vi "Read Action.vi"(8 "error in (no error)":errorcluster, 11 "Debug Data in":refnum<class "Debug Data.lvclass">) -> (0 "error out":errorcluster, 2 "Action":string, 3 "Debug Data out":refnum<class "Debug Data.lvclass">)   [LabVIEW 2020, in "Debug Data.lvclass"]
uses:
  Debug Data.lvclass
  Debug Data.lvclass/Debug Data.ctl
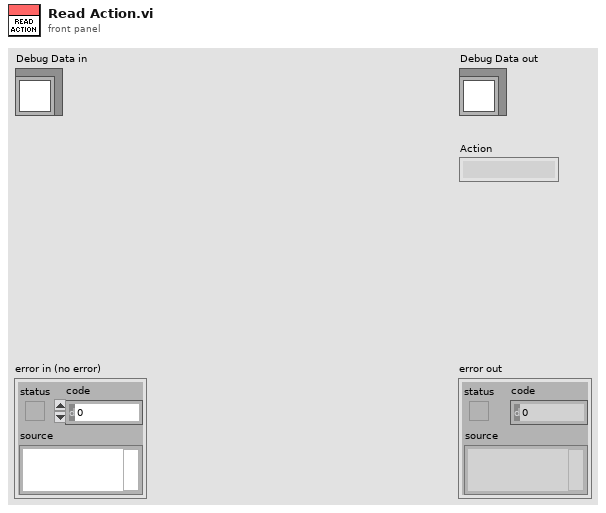
[diagram p1: front panel]
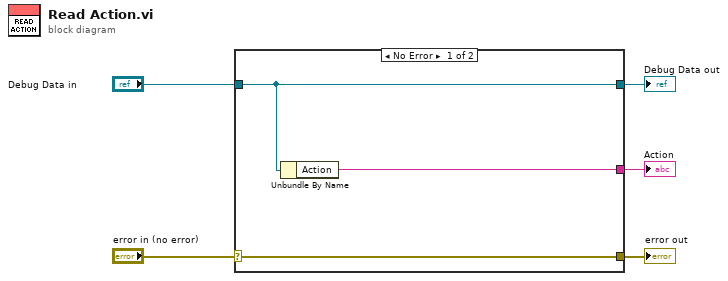
[diagram p0: block diagram]
diagram:
  n1 = case shown="No Error" "error in (no error)" {
    selector: "error in (no error)" -> [w8 w9]
    tunnel: [w8 w9] -> w4
    tunnel: [w7 w10] -> w2
    tunnel: "Debug Data in" -> [w7 w10]
    tunnel: [w6 _] -> w1
    frame No Error {
      n2 = Unbundle By Name(w7) -> ("Action"=w6:string)
    }
    frame Error {
    }
  }
  "error out" <- w4
  "Debug Data out" <- w2
  "Action" <- w1
